vi "RT-Main (lunch only).vi"() -> ()   [LabVIEW 2016]
uses:
  <vilib>/NI_Real-Time Target Support.lvlib
panel:
  in  "Stop Button":bool
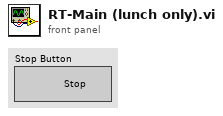
[diagram p1: front panel]
types:
  T1 = typedef "Array AE Data.ctl" = T2[]
  T2 = typedef "AE Data.ctl" = cluster{"Name":string, "Go?":bool, "Which batch?":enum16{"Anything", "First", "Second"}}
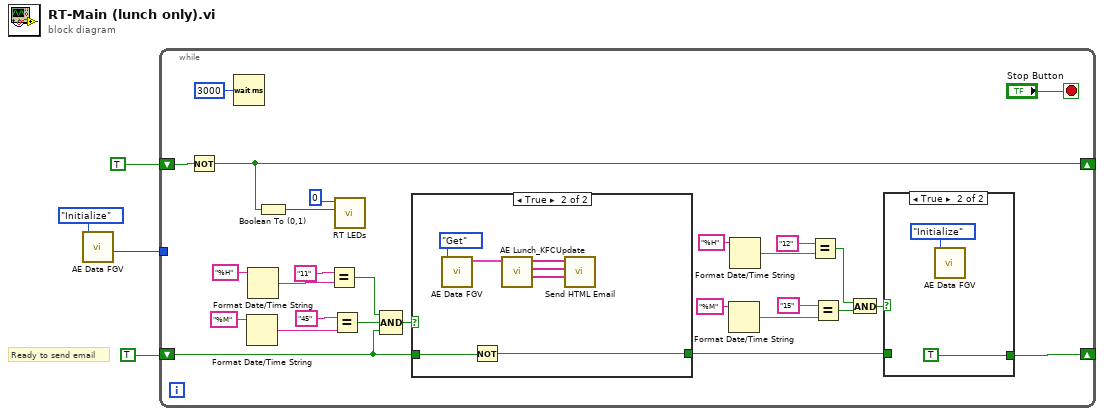
[diagram p0: block diagram]
diagram:
  # "Ready to send email"
  n1 = call "AE Data FGV.vi"("Command"=enum16{"Initialize", "Update", "Get"}."Initialize") -> ("Index"=w1:i32)  [unwired: 9 in, 1 out]
  n2 = while {
    shift-right: [w29] -> _
    shift-left: TRUE -> [w30]
    shift-right: [w5] -> _
    shift-left: TRUE -> [w16]
    tunnel: w1 -> [_]
    stop <- "Stop Button" stop-if-true
    n3 = Not(x=w30) -> (.not. x?=w29:bool)
    n4 = Wait (ms)(milliseconds to wait=u32 3000) -> ()  [unwired: 1 out]
    n5 = Format Date/Time String(time format string (%c)="%M") -> (date/time string=w21:string)  [unwired: 2 in]
    n6 = Format Date/Time String(time format string (%c)="%H") -> (date/time string=w23:string)  [unwired: 2 in]
    n7 = Boolean To (0,1)(Boolean=w29) -> (0, 1=w28:i16)
    n8 = Equal?(x="11", y=w23) -> (x = y?=w19:bool)
    n9 = Equal?(x="45", y=w21) -> (x = y?=w18:bool)
    n10 = call <vilib>:"RT LEDs.vi"("State"=w28, "LED Num"=0) -> ()  [unwired: 4 in, 2 out]
    n11 = Compound Arithmetic op=AND(w19, w18, w16) -> (w17:bool)
    n12 = case shown="True" w17 {
      tunnel: w16 -> [w32 w39]
      tunnel: [w32 w38] -> w6
      frame False {
      }
      frame True {
        n13 = call "AE Data FGV.vi"("Command"=enum16{"Initialize", "Update", "Get"}."Get") -> ("Array of AEs"=w36:T1)  [unwired: 9 in, 1 out]
        n14 = Not(x=w39) -> (.not. x?=w38:bool)
        n15 = call "AE Lunch_KFCUpdate.vi"("Array of AEs"=w36) -> ("Not Going"=w33:string[], "Second Batch"=w34:string[], "First Batch"=w35:string[])  [unwired: 8 in]
        n16 = call "Send HTML Email.vi"("Not Going"=w33, "Second Batch"=w34, "First Batch"=w35) -> ()  [unwired: 7 in, 2 out]
      }
    }
    n17 = Format Date/Time String(time format string (%c)="%M") -> (date/time string=w14:string)  [unwired: 2 in]
    n18 = Format Date/Time String(time format string (%c)="%H") -> (date/time string=w12:string)  [unwired: 2 in]
    n19 = Equal?(x="12", y=w12) -> (x = y?=w9:bool)
    n20 = Equal?(x="15", y=w14) -> (x = y?=w8:bool)
    n21 = And(x=w9, y=w8) -> (x .and. y?=w7:bool)
    n22 = case shown="True" w7 {
      tunnel: w6 -> [w40 _]
      tunnel: [w40 TRUE] -> w5
      frame False {
      }
      frame True {
        n23 = call "AE Data FGV.vi"("Command"=enum16{"Initialize", "Update", "Get"}."Initialize") -> ()  [unwired: 9 in, 2 out]
      }
    }
  }
